vi "SaveData.vi"(7 "ThisVI_In":refnum<vi>, 9 "Main menu in":refnum<vi>, 11 "Output Values of Device":refnum<vi>) -> (1 "Main menu out":refnum<vi>)   [LabVIEW 2013]
panel:
  out "error out":errorcluster
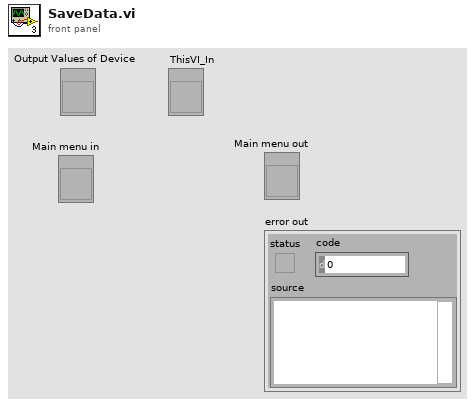
[diagram p1: front panel]
types:
  T1 = cluster{"Measurement":bool, "Save Data":bool, "LoadSetting":bool, "Save setting":bool, "Reset setting":bool, "Exit":bool}
  T2 = enum16{"open", "replace", "create", "open or create", "replace or create", "replace or create with confirmation"}
  T3 = cluster{"KEITHLEY 2182 & KEITHLEY 6221":dbl[][], "Other Devices":dbl[][]}
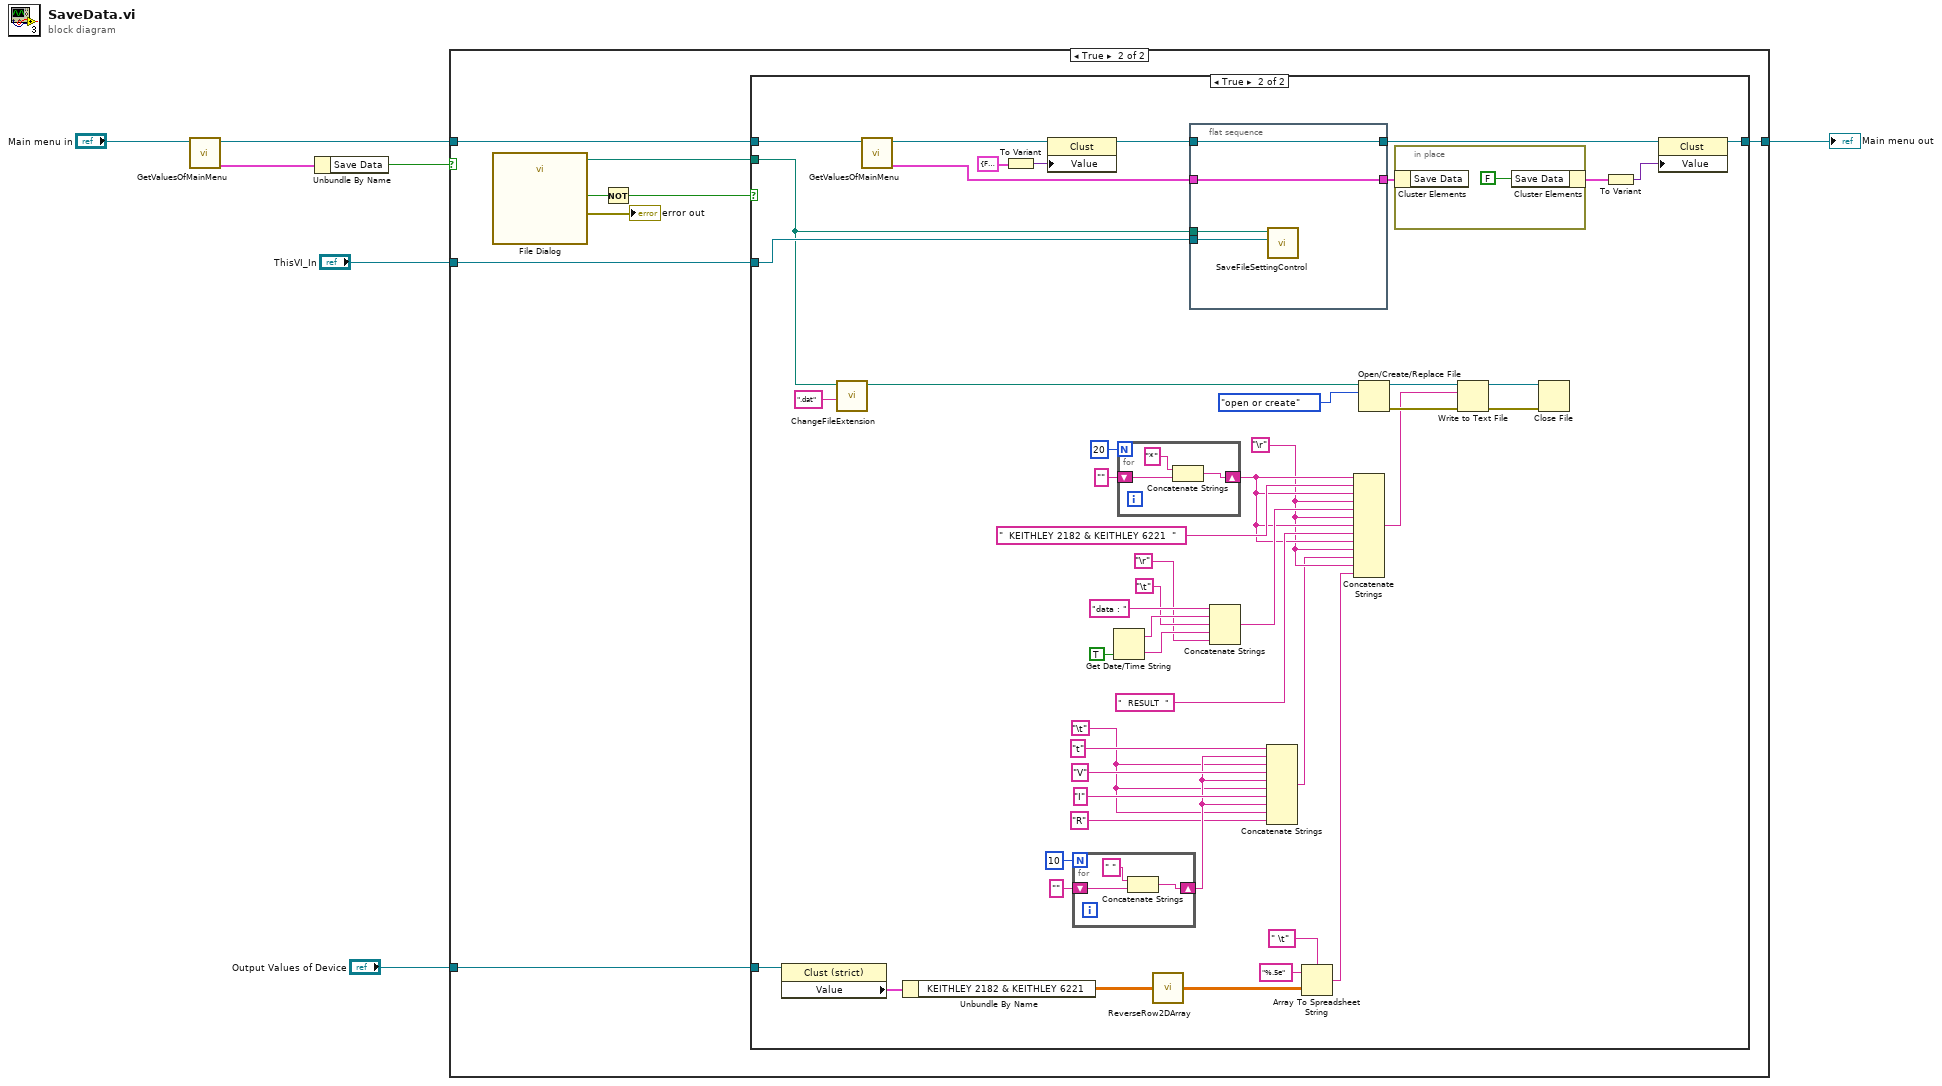
[diagram p0: block diagram]
diagram:
  n1 = call "GetValuesOfMainMenu.vi"("MainMenu_In"="Main menu in") -> ("ValuesOfMainMenu"=w6:T1, "MainMenu_Out"=w2:refnum<vi>)  [unwired: 9 in]
  n2 = Unbundle By Name(w6) -> ("Save Data"=w5:bool)
  n3 = case shown="True" w5 {
    tunnel: "Output Values of Device" -> [_ w9]
    tunnel: "ThisVI_In" -> [_ w13]
    tunnel: w2 -> [w8 w11]
    tunnel: [w8 w10] -> w1
    frame False {
    }
    frame True {
      n4 = call "File Dialog"() -> ("selected path"=w14:path, "cancelled"=w16:bool, "error out"=→"error out":errorcluster)  [unwired: 12 in, 1 out]
      n5 = Not(x=w16) -> (.not. x?=w15:bool)
      n6 = case shown="True" w15 {
        tunnel: w14 -> [_ w54]
        tunnel: w13 -> [_ w60]
        tunnel: w11 -> [w17 w65]
        tunnel: [w17 w61] -> w10
        tunnel: w9 -> [_ w34]
        frame False {
        }
        frame True {
          w22 = "\t"
          w30 = "\r"
          n7 = property class="Clust (strict)"(reference=w34) -> ("Value"=w33:T3)  [unwired: 1 in, 2 out]
          n8 = call "ChangeFileExtension.vi"("NewFileExtension"=".dat", "Path to was selected by user"=w54) -> ("appended path"=w53:path)  [unwired: 9 in]
          n9 = call "GetValuesOfMainMenu.vi"("MainMenu_In"=w65) -> ("ValuesOfMainMenu"=w57:T1, "MainMenu_Out"=w64:refnum<vi>)  [unwired: 9 in]
          n10 = Unbundle By Name(w33) -> ("KEITHLEY 2182 & KEITHLEY 6221"=w19:dbl[][])
          n11 = To Variant(anything=T1 {"Measurement"=FALSE, "Save Data"=FALSE, "LoadSetting"=FALSE, "Save setting"=FALSE, "Reset setting"=FALSE, "Exit"=FALSE} ("Main menu")) -> (Variant=w67:variant)
          n12 = property class="Clust"(reference=w64, "Value"=w67) -> (reference out=w58:refnum<vi>)  [unwired: 1 in, 1 out]
          n13 = for {
            N: 10 -> [_]
            shift-right: [w70] -> w23
            shift-left: "" -> [w69]
            n14 = Concatenate Strings(" ", w69) -> (w70:string)
          }
          n15 = Get Date/Time String(want seconds? (F)=TRUE) -> (date string=w46:string, time string=w44:string)  [unwired: 2 in]
          n16 = for {
            N: 20 -> [_]
            shift-right: [w73] -> w40
            shift-left: "" -> [w72]
            n17 = Concatenate Strings("*", w72) -> (w73:string)
          }
          n18 = call "ReverseRow2DArray.vi"("2DArray_in"=w19) -> ("2DArray_out"=w18:dbl[][])
          n19 = flat-sequence {
            tunnel: w54 -> [w77]
            tunnel: w60 -> [w76]
            tunnel: [w75] -> w59
            tunnel: w58 -> [w75]
            tunnel: w57 -> [w74]
            tunnel: [w74] -> w56
            frame #0 {
              n20 = call "SaveFileSettingControl.vi"("This VI"=w76, "Path to was selected by user"=w77) -> ()  [unwired: 9 in, 1 out]
            }
          }
          n21 = Concatenate Strings("data : ", w46, "\t", w44, "\r") -> (w42:string)
          n22 = Concatenate Strings("t", w23, w22, "V", w23, w22, "I", w23, w22, "R") -> (w20:string)
          n23 = Array To Spreadsheet String(delimiter (Tab)=" \t", array=w18, 3:"%.5e" ("format string")) -> (spreadsheet string=w31:string)
          n24 = Concatenate Strings(w40, "  KEITHLEY 2182 & KEITHLEY 6221  ", w40, w30, w42, w30, w40, "  RESULT  ", w40, w30, w20, w30, w31) -> (w35:string)
          n25 = Open/Create/Replace File(file path (use dialog)=w53, operation (0:open)=T2."open or create") -> (refnum out=w39:refnum<file>, error out=w37:errorcluster)  [unwired: 4 in, 1 out]
          n26 = in-place {
            n27 = in-place-cluster #1(w56) -> ()  [unwired: 1 out]
            n28 = in-place-cluster #1("Save Data"=FALSE) -> (w63:T1)
          }
          n29 = Write to Text File(file (use dialog)=w39, text=w35, error in=w37) -> (refnum out=w38:refnum<file>, error out=w36:errorcluster)  [unwired: 1 in, 1 out]
          n30 = Close File(refnum=w38, error in=w36) -> ()  [unwired: 2 out]
          n31 = To Variant(anything=w63) -> (Variant=w62:variant)
          n32 = property class="Clust"(reference=w59, "Value"=w62) -> (reference out=w61:refnum<vi>)  [unwired: 1 in, 1 out]
        }
      }
    }
  }
  "Main menu out" <- w1
